vi "Add Custom Device Section - Offline.vi"(4 "Property Values":variant[](array[variant]), 5 "Highlight? (F)":bool, 6 "Property names":string[](array[string]), 7 "GUID (Default Section)":string="03D3BB89-1485-13A6-56005DE6430FF8B7", 8 "error in (no error)":errorcluster, 10 "Section Name":string, 11 "Parent Ref in":T1 format="%.0x") -> (0 "error out":errorcluster, 1 "Section Ptr":T1 format="%.0x", 2 "Newly Created?":bool, 3 "Parent Ref out":T1 format="%.0x")   [LabVIEW 2020, in "Ballard Arinc-429 System Explorer.lvlib"]
uses:
  Ballard Arinc-429 System Explorer.lvlib
  <vilib>/NI VeriStand/Custom Device Offline API/Custom Device Offline API.lvlib
  NationalInstruments.VeriStand.SystemDefinitionAPI
  <vilib>/NI VeriStand/Custom Device API/Custom Device Item Ref.ctl
  <vilib>/NI VeriStand/Custom Device API/Custom Device API.lvlib
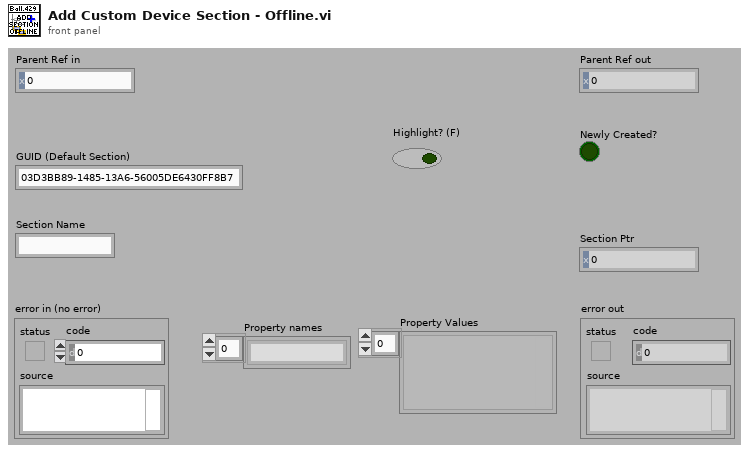
[diagram p1: front panel]
types:
  T1 = typedef "Custom Device API.lvlib/Custom Device Item Ref.ctl" = u64
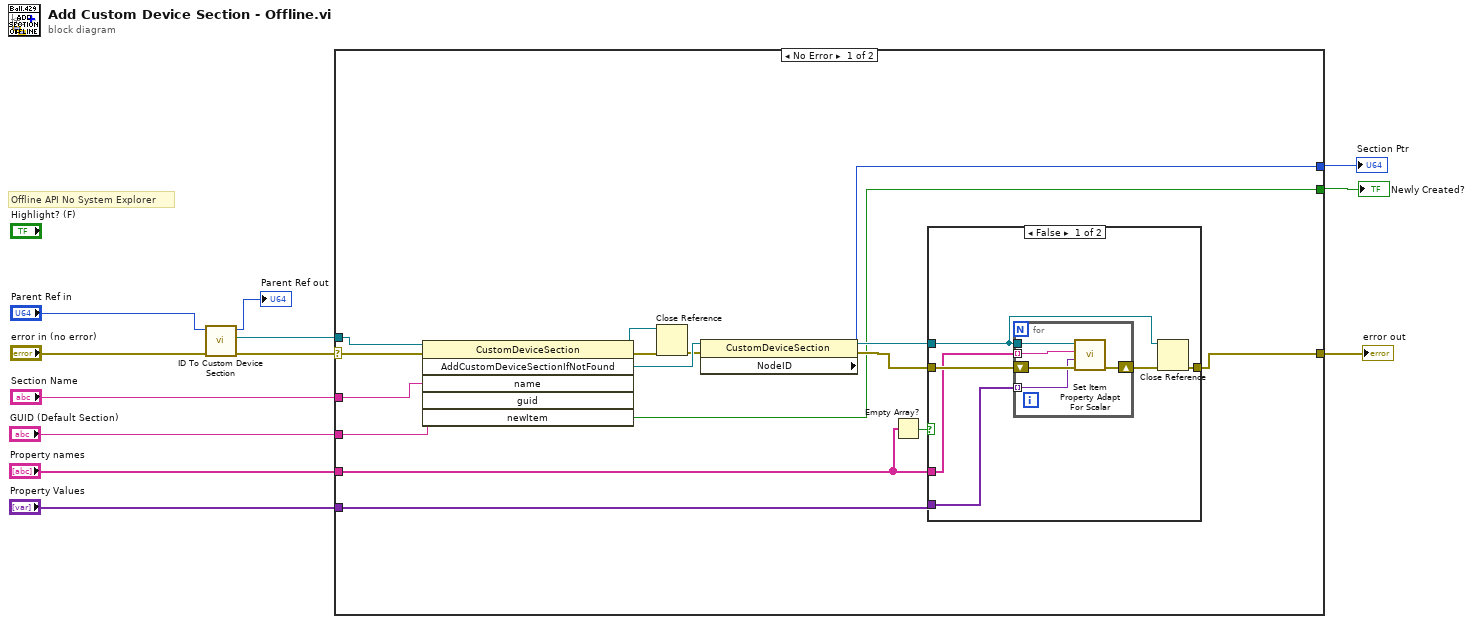
[diagram p0: block diagram]
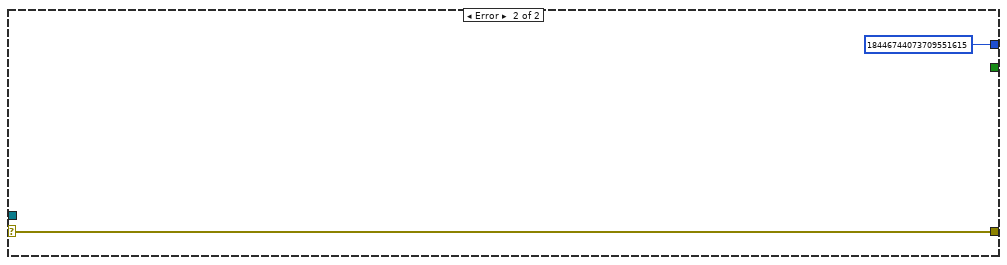
[diagram p3: hidden frame]
diagram:
  # "Offline API No System Explorer"
  n1 = call <vilib>:"ID To Custom Device Section.vi"("error in (no error)"="error in (no error)", "ID in"="Parent Ref in") -> ("error out"=w11:errorcluster, "Section"=w9:refnum<k24>, "ID out"=→"Parent Ref out":u64)  [unwired: 7 in]
  n2 = case shown="No Error" w11 {
    selector: w11 -> [w27 w42]
    tunnel: [w24 w42] -> w10
    tunnel: w9 -> [w28 _]
    tunnel: "Section Name" -> [w26 _]
    tunnel: "GUID (Default Section)" -> [w25 _]
    tunnel: [w19 T1 18446744073709551615 ("Section Ptr")] -> w4
    tunnel: [w16 _] -> w3
    tunnel: "Property names" -> [w15 _]
    tunnel: "Property Values" -> [w14 _]
    frame No Error {
      n3 = invoke class="CustomDeviceSection" method="AddCustomDeviceSectionIfNotFound"(reference=w28, error in=w27, "name"=w26, "guid"=w25) -> (reference out=w22:refnum<k24>, error out=w23:errorcluster, "AddCustomDeviceSectionIfNotFound"=w21:refnum<k24>, "newItem"=w16:bool)  [unwired: 2 in, 2 out]
      n4 = Close Reference(reference=w22, error in (no error)=w23) -> (error out=w20:errorcluster)
      n5 = property class="CustomDeviceSection"(reference=w21, error in=w20) -> (reference out=w17:refnum<k24>, error out=w18:errorcluster, "NodeID"=w19:u64)
      n6 = Empty Array?(array=w15) -> (empty?=w13:bool)
      n7 = case shown="False" w13 {
        tunnel: w17 -> [w30 _]
        tunnel: w18 -> [w34 w40]
        tunnel: w14 -> [w33 _]
        tunnel: w15 -> [w32 _]
        tunnel: [w29 w40] -> w24
        frame False {
          n8 = for {
            tunnel: w33 -> [w38] mode=indexing
            tunnel: w32 -> [w37] mode=indexing
            shift-right: [w35] -> w31
            shift-left: w34 -> [w39]
            tunnel: w30 -> [w36]
            n9 = call <vilib>:"Set Item Property Adapt For Scalar.vi"("error in (no error)"=w39, "Value"=w38, "Property Name"=w37, "CDBase"=w36) -> ("error out"=w35:errorcluster)  [unwired: 5 in, 2 out]
          }
          n10 = Close Reference(reference=w30, error in (no error)=w31) -> (error out=w29:errorcluster)
        }
        frame True {
        }
      }
    }
    frame Error {
    }
  }
  "error out" <- w10
  "Section Ptr" <- w4
  "Newly Created?" <- w3
